vi "SRP_Socket_ReadWrite.vi"(7 "error in (no error)":errorcluster, 10 "Data In":string) -> (0 "error out":errorcluster, 3 "Data Out":string)   [LabVIEW 2011]
doc: "This VI writes and reads to the SRP socket.\n\nInputs:\n1. Data In: Command to sent to SRP socket (do script, int variable, getVar etc.)\n\nOutputs:\n1. Data Out: SRP socket response (OK, Error, getVar value, etc.)"
uses:
  <vilib>/Utility/error.llb/DialogType.ctl
  Global_SRP_Socket.vi
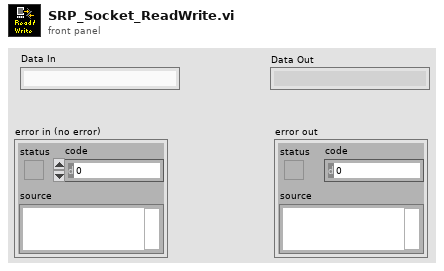
[diagram p1: front panel]
types:
  T1 = enum16{"Standard", "Buffered", "CRLF", "Immediate"}
  T2 = typedef "DialogType.ctl" = u16
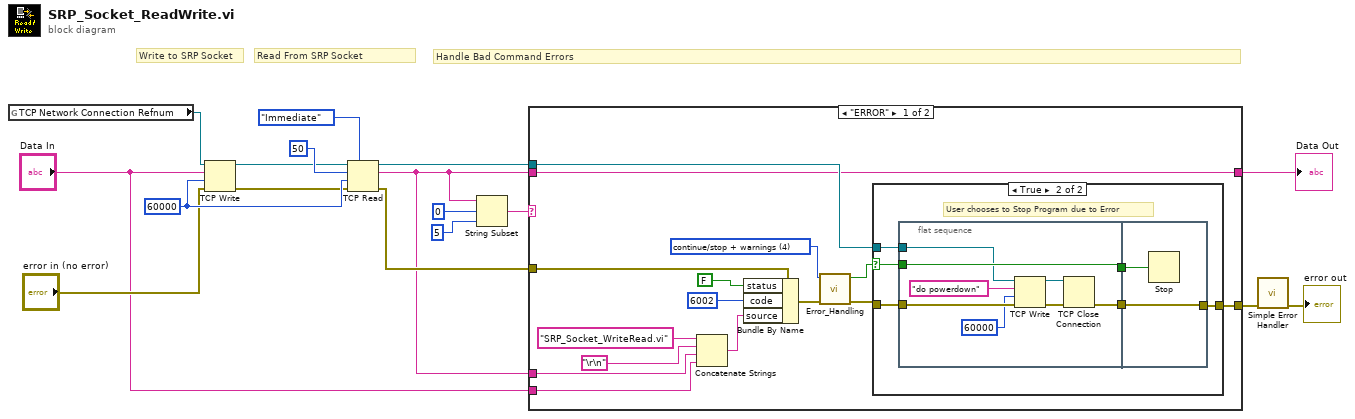
[diagram p0: block diagram]
diagram:
  w17 = 60000 ("timeout ms (60000)")
  # "Handle Bad Command Errors"
  # "Read From SRP Socket"
  # "Write to SRP Socket"
  n1 = global read "Global_SRP_Socket.vi" "TCP Network Connection Refnum"() -> (w13:refnum<k5>)
  n2 = TCP Write(connection ID=w13, data in="Data In", error in (no error)="error in (no error)", 9:w17) -> (connection ID out=w14:refnum<k5>, error out=w11:errorcluster)  [unwired: 1 out]
  n3 = TCP Read(connection ID=w14, bytes to read=50, error in (no error)=w11, 7:T1."Immediate" ("mode (standard)"), 9:w17) -> (connection ID out=w6:refnum<k5>, data out=w2:string, error out=w7:errorcluster)
  n4 = String Subset(string=w2, offset (0)=0, length (rest)=5 ("length (rest)")) -> (substring=w8:string)
  n5 = case shown="\"ERROR\"" w8 {
    tunnel: w7 -> [w25 w51]
    tunnel: w6 -> [w32 _]
    tunnel: [w31 w51] -> w4
    tunnel: [w30 w50] -> w5
    tunnel: w2 -> [w30 w50]
    tunnel: w2 -> [w21 _]
    tunnel: "Data In" -> [w20 _]
    frame "ERROR" {
      w19 = T2 4 items=["no dialog", "OK message", "continue or stop message", "OK message + warnings", "continue/stop + warnings"] ("type of dialog (OK msg:1)")
      n6 = Concatenate Strings("SRP_Socket_WriteRead.vi", "\r\n", w21, w20) -> (w26:string)
      n7 = Bundle By Name(cluster=w25, "status"=FALSE, "code"=6002, "source"=w26) -> (w29:errorcluster)
      n8 = call "Error_Handling.vi"("error in (no error)"=w29, "type of dialog (OK msg:1)"=w19) -> ("error out"=w24:errorcluster, "error?"=w18:bool)  [unwired: 8 in]
      n9 = case shown="True" w18 {
        selector: w18 -> [_ w35]
        tunnel: w24 -> [w33 w39]
        tunnel: [w33 w37] -> w31
        tunnel: w32 -> [_ w34]
        frame False {
          # "Continue Despire Error"
        }
        frame True {
          # "User chooses to Stop Program due to Error"
          n10 = flat-sequence {
            tunnel: w39 -> [w44]
            tunnel: [w47] -> w38
            tunnel: [w46] -> w36
            tunnel: w35 -> [w46]
            tunnel: w34 -> [w42]
            tunnel: [w49] -> w37
            tunnel: w38 -> [w49]
            tunnel: w36 -> [w48]
            frame #0 {
              n11 = TCP Write(connection ID=w42, data in="do powerdown", error in (no error)=w44, 9:60000 ("timeout ms (25000)")) -> (connection ID out=w43:refnum<k5>, error out=w45:errorcluster)  [unwired: 1 out]
              n12 = TCP Close Connection(connection ID=w43, error in (no error)=w45) -> (error out=w47:errorcluster)  [unwired: 1 in, 1 out]
            }
            frame #1 {
              n13 = Stop(stop? (T)=w48) -> ()
            }
          }
        }
      }
    }
    frame "OK   ", Default {
      # "This case accounts for good commands (\"OK\") and getVar values."
    }
  }
  "Data Out" <- w5
  n14 = call <vilib>:"Simple Error Handler.vi"("error in (no error)"=w4) -> ("error out"=→"error out":errorcluster)  [unwired: 4 in, 4 out]
